vi "FacadeResizable2DArray(I64).vi"(0 "Data In":T4, 2 "Display State In":T2, 3 "Container State":T3) -> (6 "Data Out":T4, 7 "Display State Out":T2, 8 "Action":T1)   [LabVIEW 2011, in "Resizable2DArray(I64).xctl"]
uses:
  <vilib>/_probes/SAPHIR/ViBox - Probes/Resizable2DArray/Resizable2DArray(I64)/Resizable2DArray(I64).xctl
  <vilib>/_probes/SAPHIR/ViBox - Probes/Resizable2DArray/Resizable2DArray(I64)/DataResizable2DArray(I64).ctl
  <vilib>/_xctls/Container State.ctl
  <vilib>/_probes/SAPHIR/ViBox - Probes/Resizable2DArray/Resizable2DArray(I64)/StateResizable2DArray(I64).ctl
  <vilib>/_xctls/Action.ctl
  <vilib>/_xctls/XControlSupport.lvlib
panel:
  in  "Format":string caption="Format :"
  out "Numeric":i64
  out "[I64]":i64[][](array[numeric])
  # "Display Options"
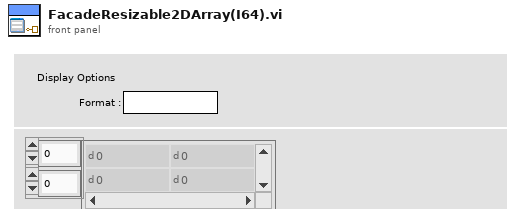
[diagram p1: front panel]
types:
  T1 = typedef "XControlSupport.lvlib/Action.ctl" = cluster{"Data Changed?":bool, "State Changed?":bool, "Action Name":string}
  T2 = typedef "Resizable2DArray(I64).xctl/StateResizable2DArray(I64).ctl" = cluster{"Height":u32, "Width":u32, "TextWidth":u32}
  T3 = typedef "XControlSupport.lvlib/Container State.ctl" = cluster{"Indicator?":bool, "Run Mode?":bool, " Refnum":refnum<vi>}
  T4 = typedef "Resizable2DArray(I64).xctl/DataResizable2DArray(I64).ctl" = i64[][]
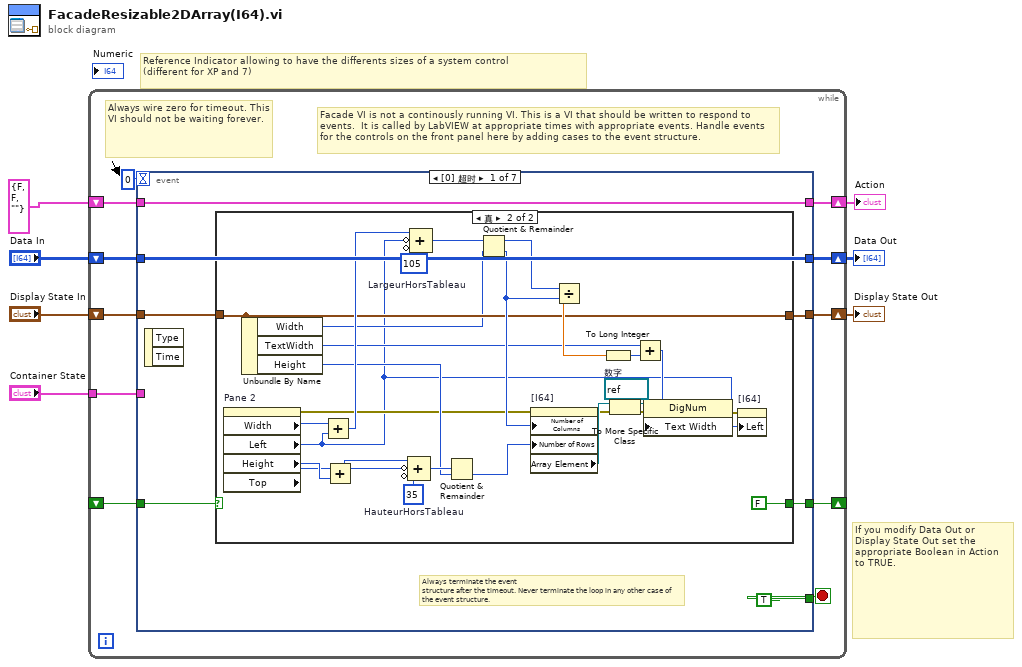
[diagram p0: block diagram]
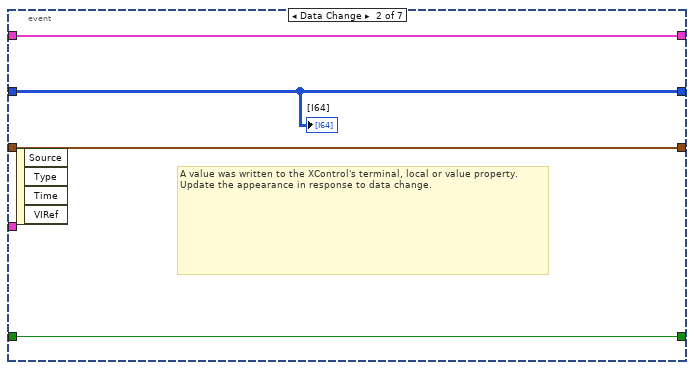
[diagram p3: hidden frame]
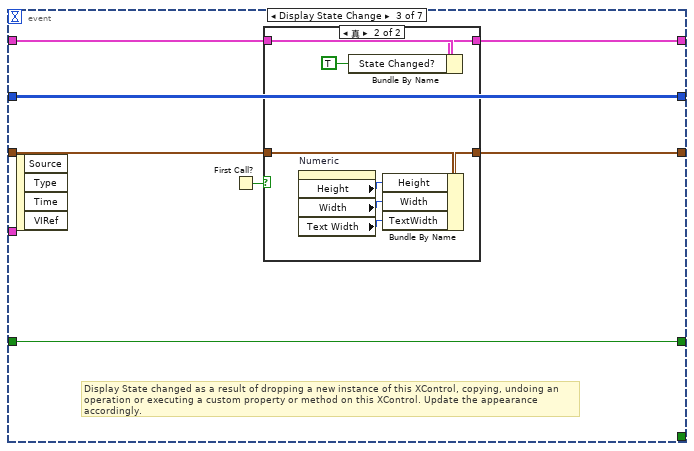
[diagram p4: hidden frame]
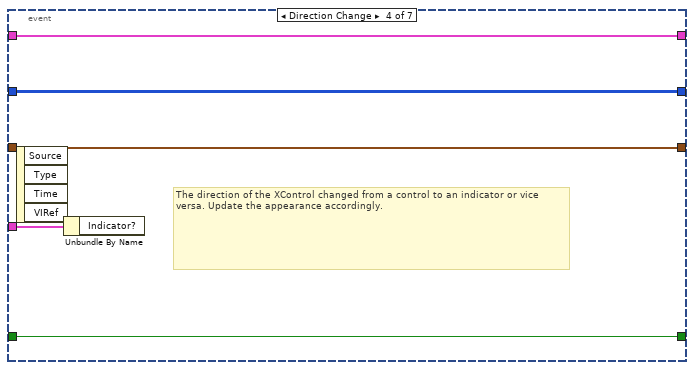
[diagram p6: hidden frame]
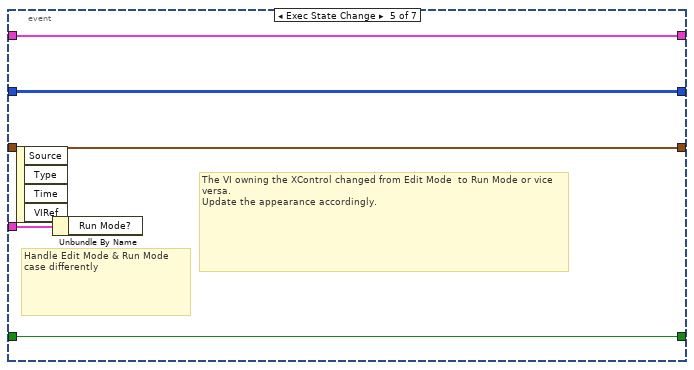
[diagram p7: hidden frame]
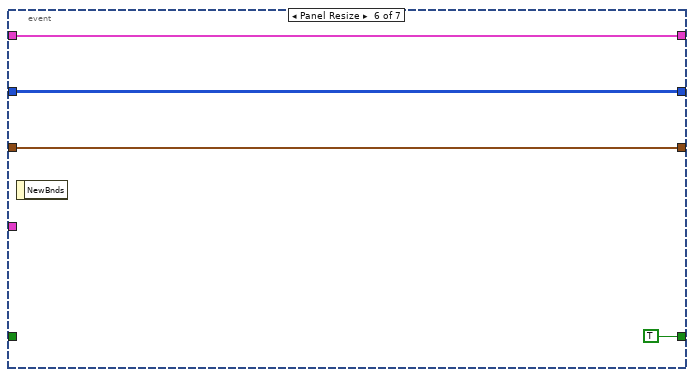
[diagram p8: hidden frame]
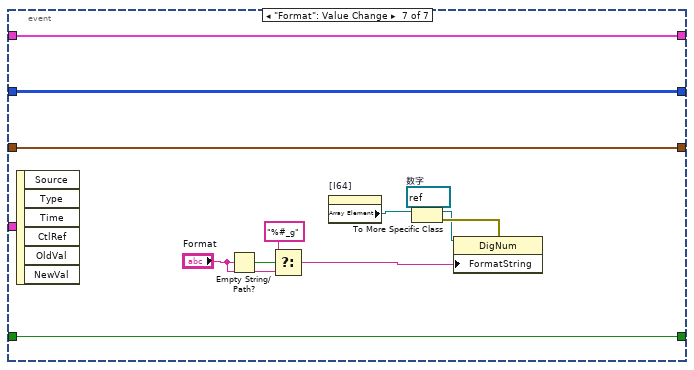
[diagram p9: hidden frame]
diagram:
  # "Reference Indicator allowing to have the differents sizes of a system control\n(different for XP and 7)"
  # "If you modify Data Out or\nDisplay State Out set the\nappropriate Boolean in Action\nto TRUE."
  n1 = while {
    shift-right: [w17] -> w5
    shift-left: "Display State In" -> [w18]
    tunnel: "Container State" -> [w14]
    shift-right: [w12] -> w7
    shift-left: "Data In" -> [w13]
    shift-right: [w10] -> w3
    shift-left: T1 {"Data Changed?"=FALSE, "State Changed?"=FALSE, "Action Name"=""} ("Action") -> [w11]
    shift-right: [w8] -> _
    shift-left: _ -> [w9]
    stop <- w16 stop-if-true
    # "Facade VI is not a continously running VI. This is a VI that should be written to respond to events.  It is called by LabVIEW at appropriate times with appropriate events. Handle events for the controls on the front panel here by adding cases to the event structure."
    # "Always wire zero for timeout. This\nVI should not be waiting forever."
    n2 = event shown="[0] 超时" {
      selector: _ -> [_ _ _ _ _ _ _]
      dyn-events: _ -> [_ _ _ _ _ _ _]
      timeout: 0 -> [_ _ _ _ _ _ _]
      tunnel: w18 -> [w22 w59 w61 w80 w85 w88 w99]
      tunnel: [w19 w59 w60 w80 w85 w88 w99] -> w17
      tunnel: [TRUE _ _ _ _ _ _] -> w16
      tunnel: w14 -> [_ _ _ w81 w86 _ _]
      tunnel: w13 -> [w23 w57 w66 w79 w84 w90 w100]
      tunnel: [w23 w57 w66 w79 w84 w90 w100] -> w12
      tunnel: [w24 w58 w62 w78 w83 w89 w101] -> w10
      tunnel: w11 -> [w24 w58 w63 w78 w83 w89 w101]
      tunnel: w9 -> [w21 w56 w65 w77 w82 _ w102]
      tunnel: [w20 w56 w65 w77 w82 TRUE w102] -> w8
      event Timeout {
        # "Always terminate the event\nstructure after the timeout. Never terminate the loop in any other case of the event structure."
        n3 = event-data() -> ()  [unwired: 3 out]
        n4 = case shown="真" w21 {
          selector: w21 -> [w27 _]
          tunnel: w22 -> [w26 w36]
          tunnel: [w27 FALSE] -> w20
          tunnel: [w26 w36] -> w19
          frame False {
          }
          frame True {
            w51 = refnum<vi> refnum  # 数字
            w53 = i16 35  # HauteurHorsTableau
            w52 = i16 105  # LargeurHorsTableau
            n5 = property on="Pane 2" class="Pane"() -> (error out=w32:errorcluster, "Width"=w31:u32, "Left"=w30:i32, "Height"=w29:u32, "Top"=w28:i32)  [unwired: 2 in, 1 out]
            n6 = Unbundle By Name(w36) -> ("Width"=w35:u32, "TextWidth"=w34:u32, "Height"=w33:u32)
            n7 = Add(x=w31, y=w30) -> (x+y=w54:u32)
            n8 = Add(x=w28, y=w29) -> (x+y=w40:u32)
            n9 = Compound Arithmetic op=ADD(w40, invert w28, invert w53) -> (w44:u32)
            n10 = Compound Arithmetic op=ADD(w54, invert w30, invert w52) -> (w48:u32)
            n11 = Quotient & Remainder(x=w44, y=w33) -> (floor(x/y)=w38:u32)  [unwired: 1 out]
            n12 = Quotient & Remainder(x=w48, y=w35) -> (x-y*floor(x/y)=w55:u32, floor(x/y)=w39:u32)
            n13 = property on="[I64]" class="Arr (严格)"(error in=w32, "Number of Columns"=w39, "Number of Rows"=w38) -> (error out=w43:errorcluster, "Array Element"=w45:refnum<vi>)  [unwired: 1 in, 1 out]
            n14 = Divide(x=w55, y=w39) -> (x/y=w47:dbl)
            n15 = To Long Integer(number=w47) -> (32bit integer=w46:i32)
            n16 = To More Specific Class(target class=w51, reference=w45, error in=w43) -> (specific class reference=w50:refnum<vi>, error out=w42:errorcluster)
            n17 = Add(x=w34, y=w46) -> (x+y=w49:u32)
            n18 = property class="DigNum"(reference=w50, error in=w42, "Text Width"=w49) -> (error out=w41:errorcluster)  [unwired: 1 out]
            n19 = property on="[I64]" class="Arr (严格)"(error in=w41, "Left"=w30) -> ()  [unwired: 1 in, 2 out]
          }
        }
      }
      event Data Change {
        # "A value was written to the XControl's terminal, local or value property.\nUpdate the appearance in response to data change."
        n20 = event-data() -> ()  [unwired: 5 out]
        "[I64]" <- w57
      }
      event Display State Change {
        # "Display State changed as a result of dropping a new instance of this XControl, copying, undoing an operation or executing a custom property or method on this XControl. Update the appearance accordingly."
        n21 = event-data() -> ()  [unwired: 5 out]
        n22 = First Call?() -> (First Call?: T/F=w64:bool)
        n23 = case shown="真" w64 {
          tunnel: w61 -> [w68 w76]
          tunnel: [w68 w75] -> w60
          tunnel: w63 -> [w67 w73]
          tunnel: [w67 w69] -> w62
          frame False {
          }
          frame True {
            n24 = property on="Numeric" class="DigNum (严格)"() -> ("Height"=w74:u32, "Width"=w71:u32, "Text Width"=w70:u32)  [unwired: 2 in, 2 out]
            n25 = Bundle By Name(cluster=w73, "State Changed?"=TRUE) -> (w69:T1)
            n26 = Bundle By Name(cluster=w76, "Height"=w74, "Width"=w71, "TextWidth"=w70) -> (w75:T2)
          }
        }
      }
      event Direction Change {
        # "The direction of the XControl changed from a control to an indicator or vice versa. Update the appearance accordingly."
        n27 = event-data() -> ()  [unwired: 5 out]
        n28 = Unbundle By Name(w81) -> ()  [unwired: 1 out]
      }
      event Exec State Change {
        # "The VI owning the XControl changed from Edit Mode  to Run Mode or vice versa.\nUpdate the appearance accordingly."
        # "Handle Edit Mode & Run Mode\ncase differently"
        n29 = event-data() -> ()  [unwired: 5 out]
        n30 = Unbundle By Name(w86) -> ()  [unwired: 1 out]
      }
      event Panel Resize {
        n31 = event-data() -> ()  [unwired: 2 out]
      }
      event "Format": Value Change {
        w92 = refnum<vi> refnum  # 数字
        n32 = event-data() -> ()  [unwired: 7 out]
        n33 = Empty String/Path?(string/path="Format") -> (empty?=w96:bool)
        n34 = Select(t="%#_g", s=w96, f="Format") -> (s? t:f=w98:string)
        n35 = property on="[I64]" class="Arr (严格)"() -> ("Array Element"=w95:refnum<vi>)  [unwired: 2 in, 2 out]
        n36 = To More Specific Class(target class=w92, reference=w95) -> (specific class reference=w93:refnum<vi>, error out=w94:errorcluster)  [unwired: 1 in]
        n37 = property class="DigNum"(reference=w93, error in=w94, "FormatString"=w98) -> ()  [unwired: 2 out]
      }
    }
  }
  "Display State Out" <- w5
  "Data Out" <- w7
  "Action" <- w3
